vi "ACCEL_TEST3.vi"() -> ()   [LabVIEW 2015]
uses:
  <vilib>/myRIO/Instrument Drivers/Onboard Devices/Accelerometer/typedefs/Accelerometer Reference.ctl
  <vilib>/myRIO/Common/Instrument Driver Framework/Utilities/typedefs/myRIO Generic Hardware Reference.ctl
  <vilib>/myRIO/Common/Instrument Driver Framework/Utilities/typedefs/Hardware Version Enum.ctl
  <vilib>/myRIO/Common/Instrument Driver Framework/Utilities/typedefs/myRIO v1.0 Reference.ctl
  <vilib>/myRIO/Common/Instrument Driver Framework/Utilities/typedefs/Generic FPGA Reference.ctl
  <vilib>/myRIO/Common/Instrument Driver Framework/myRIO v1.0/Accelerometer/typedefs/Accelerometer Channels List.ctl
  <vilib>/myRIO/Common/Instrument Driver Framework/myRIO v1.0/Accelerometer/typedefs/Accelerometer Channels Enum.ctl
  <vilib>/userdefined/High Color/nirio_resource_hc.ctl
  <vilib>/myRIO/Common/Instrument Driver Framework/Utilities/vis/Is FPGA Ref Available.vi
  <vilib>/myRIO/Common/Instrument Driver Framework/myRIO v1.0/Accelerometer/vis/myRIO v1.1 Open Accelerometer.vi
  <vilib>/myRIO/Instrument Drivers/Onboard Devices/Accelerometer/vis/Read.vi
  <vilib>/Analysis/8numeric.llb/1D Numeric Integration.vi
  <vilib>/myRIO/Common/Instrument Driver Framework/Utilities/vis/Validate Channels.vi
  <vilib>/myRIO/Common/Instrument Driver Framework/myRIO v1.0/Accelerometer/vis/myRIO v1.0 Reserve Accelerometer.vi
  <vilib>/myRIO/Common/Instrument Driver Framework/myRIO v1.0/Resource Manager/vis/myRIO v1.0 Reserve Channel List.vi
  <vilib>/myRIO/Common/Instrument Driver Framework/myRIO v1.0/Accelerometer/vis/myRIO v1.0 Build MUX Configuration Accelerometer.vi
  <vilib>/myRIO/Common/Instrument Driver Framework/myRIO v1.0/Resource Manager/vis/myRIO v1.0 Reserve Channel.vi
  <vilib>/myRIO/Common/Instrument Driver Framework/myRIO v1.0/Resource Manager/vis/myRIO v1.0 Unreserve Channel.vi
  <vilib>/myRIO/Common/Instrument Driver Framework/myRIO v1.0/Resource Manager/vis/myRIO v1.0 Build Mutex Name.vi
  <vilib>/Utility/VariantDataType/GetNumericInfo.vi
  <vilib>/Utility/error.llb/Error Cluster From Error Code.vi
  <vilib>/myRIO/Common/Instrument Driver Framework/myRIO v1.0/myRIO v1.1 Open.vi
  <vilib>/myRIO/Common/Instrument Driver Framework/myRIO v1.0/Accelerometer/vis/myRIO v1.0 Get Scaling Constant Accelerometer.vi
  <vilib>/myRIO/Common/Instrument Driver Framework/Utilities/vis/IO Manager.vi
  <vilib>/myRIO/Common/Instrument Driver Framework/Utilities/vis/Configuration Manager.vi
  <vilib>/myRIO/Common/Instrument Driver Framework/myRIO v1.0/myRIO v1.0 Close.vi
  <vilib>/myRIO/Common/Instrument Driver Framework/myRIO v1.0/Accelerometer/vis/myRIO v1.0 Read Accelerometer.vi
  <vilib>/myRIO/Express VI/Onboard Devices/Accelerometer/Accelerometer Express VI.xnode
  <vilib>/myRIO/Instrument Drivers/Onboard Devices/Accelerometer/vis/myRIO Accelerometer Open.xnode
  <vilib>/myRIO/Instrument Drivers/Onboard Devices/Accelerometer/Accelerometer.lvlib
  <vilib>/Analysis/NI_AALPro.lvlib
panel:
  in  "stop":bool
  out "X-Axis (smoothed)":dbl
  out "Waveform Chart X":dbl(graph)
  out "Waveform Chart 2":dbl(graph)
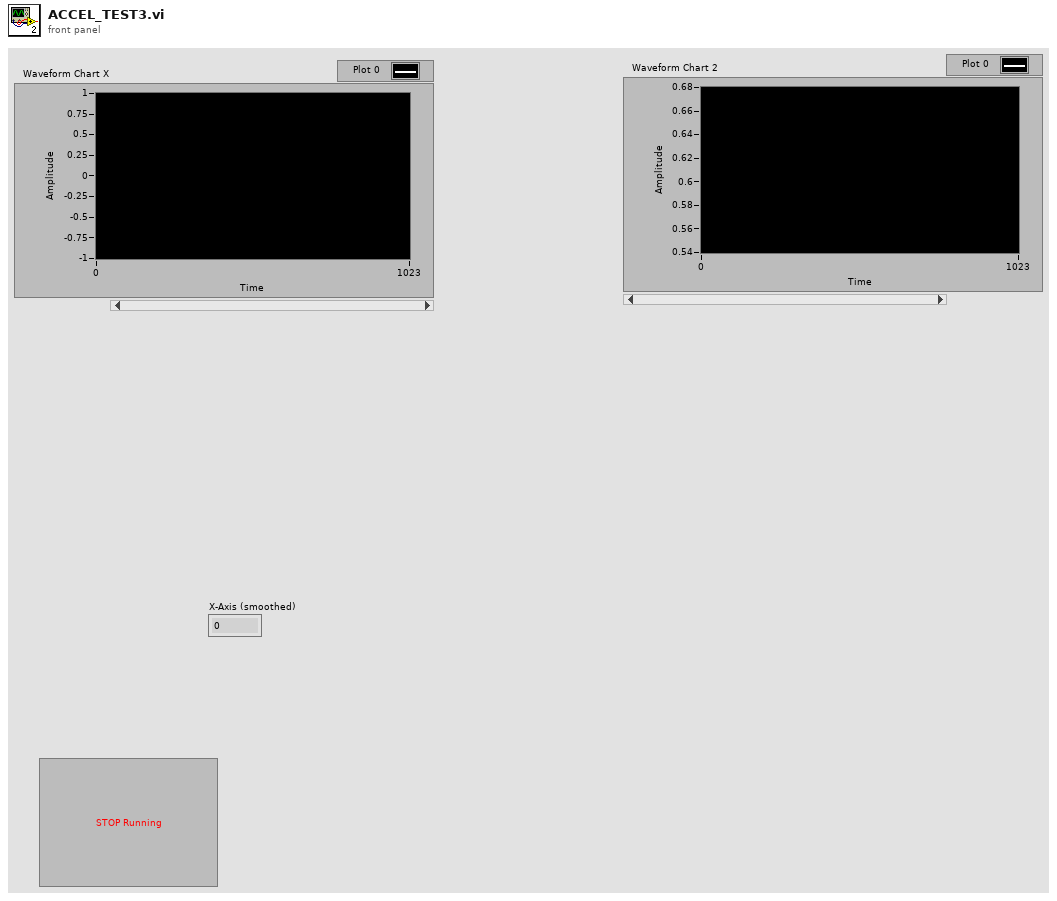
[diagram p1: front panel]
types:
  T1 = typedef "Accelerometer.lvlib/Accelerometer Reference.ctl" = cluster{"myRIO Reference":T2, "Accelerometer Channels List":T6, "LSB Weight":dbl}
  T2 = typedef "myRIO Generic Hardware Reference.ctl" = cluster{"myRIO Model":T3, "myRIO Hardware Reference":T4}
  T3 = typedef "Hardware Version Enum.ctl" = enum16{"Unknown", "myRIO-1900", "myRIO-1950", "roboRIO"}
  T4 = typedef "myRIO v1.0 Reference.ctl" = cluster{"Generic FPGA Reference":T5, "Allow multiple opens":bool}
  T5 = typedef "Generic FPGA Reference.ctl" = refnum<k20>
  T6 = typedef "Accelerometer Channels List.ctl" = T7[]
  T7 = typedef "Accelerometer Channels Enum.ctl" = enum16{"Not Connected", "X-Axis", "Y-Axis", "Z-Axis"}
  T8 = typedef "nirio_resource_hc.ctl" = tag
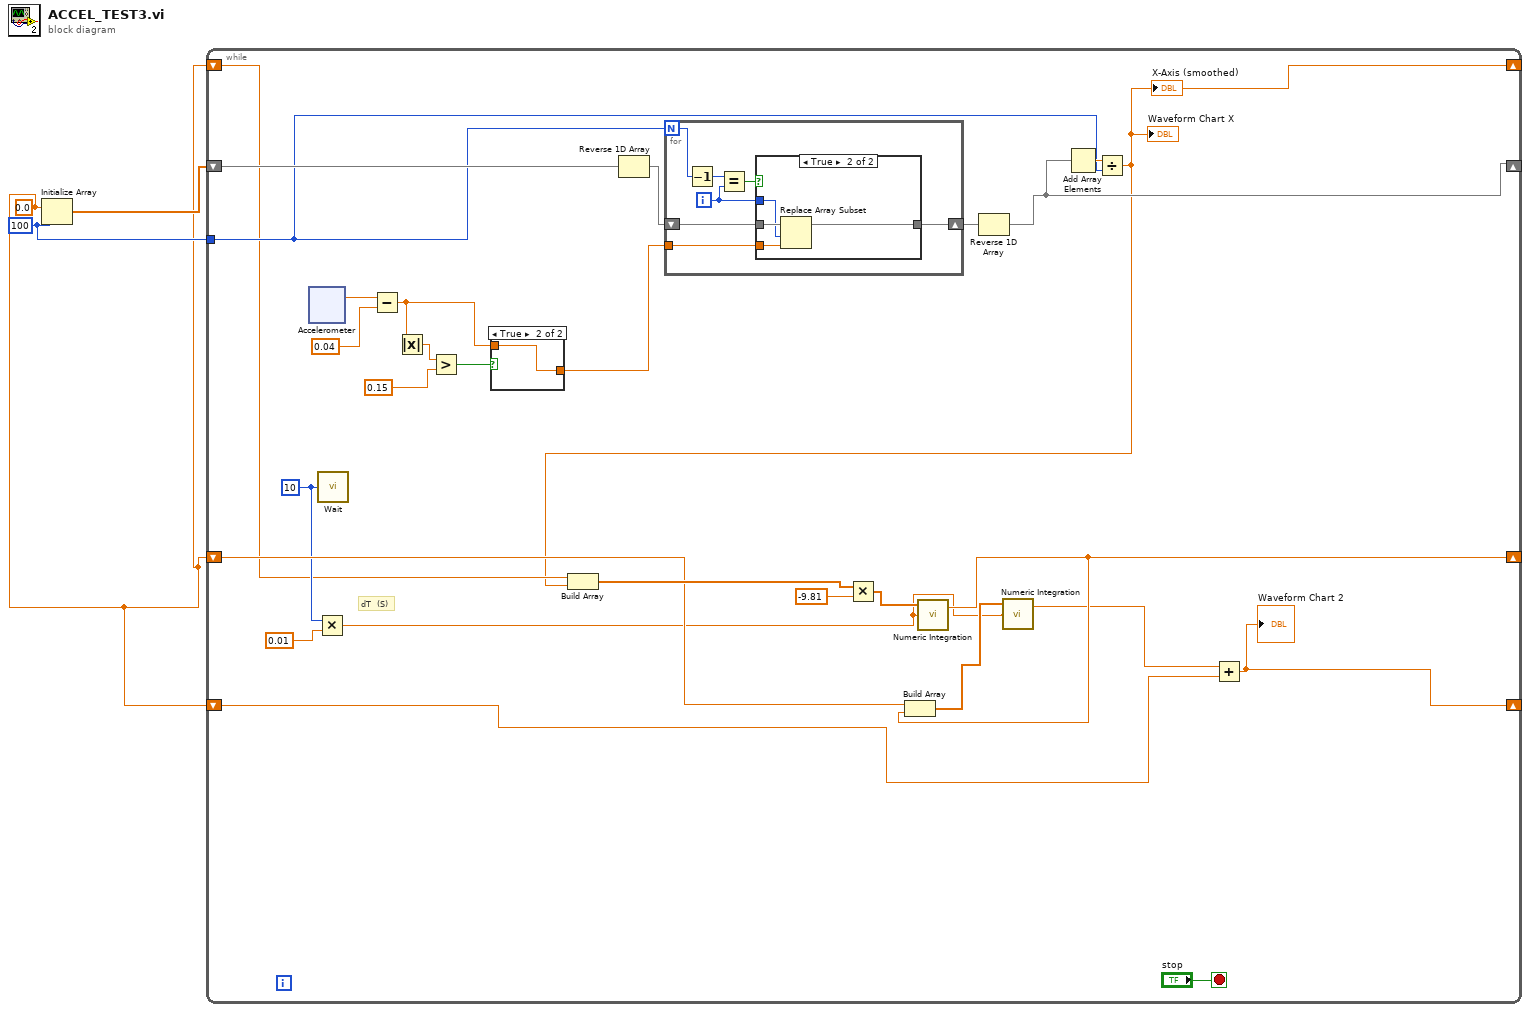
[diagram p0: block diagram]
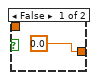
[diagram p2: hidden frame]
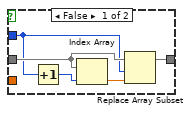
[diagram p3: hidden frame]
diagram:
  w3 = 100 ("dimension size")
  w1 = 0.0 ("element")
  n1 = Initialize Array(w1, w3) -> (w2:dbl[])
  n2 = while {
    shift-right: [w9] -> _
    shift-left: w2 -> [w27]
    tunnel: w3 -> [w11]
    shift-right: [w6] -> _
    shift-left: w1 -> [w10]
    shift-right: [w22] -> _
    shift-left: w1 -> [w23]
    shift-right: [w4] -> _
    shift-left: w1 -> [w5]
    stop <- "stop" stop-if-true
    w18 = u32 10 ("Count(mSec)")
    # "dT  (S)"
    n3 = xnode "Accelerometer"() -> ("X-Axis"=w7:dbl)  [unwired: 1 in, 2 out]
    n4 = Multiply(x=w18, y=0.01 ("element")) -> (x*y=w17:dbl)
    n5 = call "Wait"("Count(mSec)"=w18) -> ()  [unwired: 1 out]
    n6 = Subtract(x=w7, y=0.04) -> (x-y=w12:dbl)
    n7 = Absolute Value(x=w12) -> (abs(x)=w16:dbl)
    n8 = Greater?(x=w16, y=0.15) -> (0:w15:bool)
    n9 = case shown="True" w15 {
      tunnel: [0.0 ("y") w33] -> w8
      tunnel: w12 -> [_ w33]
      frame False {
      }
      frame True {
      }
    }
    n10 = Reverse 1D Array(array=w27) -> (reversed array=w30:dbl[])
    n11 = for {
      N: w11 -> [w39]
      shift-right: [w40] -> w29
      shift-left: w30 -> [w35]
      tunnel: w8 -> [w34]
      i -> [w36]
      n12 = Decrement(x=w39) -> (x-1=w37:i32)
      n13 = Equal?(x=w37, y=w36) -> (x = y?=w38:bool)
      n14 = case shown="True" w38 {
        tunnel: w36 -> [w42 w47]
        tunnel: w35 -> [w45 w48]
        tunnel: [w43 w49] -> w40
        tunnel: w34 -> [_ w46]
        frame False {
          n15 = Increment(x=w42) -> (x+1=w41:i32)
          n16 = Index Array(array=w45, index=w41) -> (element=w44:dbl)
          n17 = Replace Array Subset(array=w45, new element=w44, index=w42) -> (w43:dbl[])
        }
        frame True {
          n18 = Replace Array Subset(array=w48, new element=w46, index=w47) -> (w49:dbl[])
        }
      }
    }
    n19 = Reverse 1D Array(array=w29) -> (reversed array=w9:dbl[])
    n20 = Add Array Elements(numeric array=w9) -> (sum=w28:dbl)
    n21 = Divide(x=w28, y=w11) -> (x/y=w6:dbl)
    "X-Axis (smoothed)" <- w6
    "Waveform Chart X" <- w6
    n22 = Build Array(w10, w6) -> (w24:dbl[])
    n23 = Multiply(x=w24, y=-9.81 ("element")) -> (x*y=w25:dbl[])
    n24 = call-poly <vilib>:"Numeric Integration.vi"("dt"=w17, "Input Array"=w25) -> ("result"=w22:dbl)  [unwired: 1 in, 1 out]
    n25 = Build Array(w23, w22) -> (w21:dbl[])
    n26 = call-poly <vilib>:"Numeric Integration.vi"("dt"=w17, "Input Array"=w21) -> ("result"=w20:dbl)  [unwired: 1 in, 1 out]
    n27 = Add(x=w20, y=w5) -> (x+y=w4:dbl)
    "Waveform Chart 2" <- w4
  }
